vi "cRIO_4DoF_deactivate_mouseforce_axes.vi"(6 "Disable Yaw forces":bool, 8 "Disable X":bool, 9 "Disable Y forces":bool, 10 "Disable -X":bool, 11 "del_m in":dbl[](array[numeric])) -> (3 "del_m out":dbl[](array[numeric]))   [LabVIEW 2019]
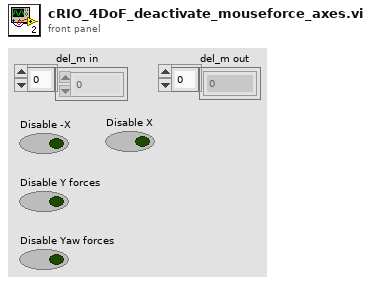
[diagram p1: front panel]
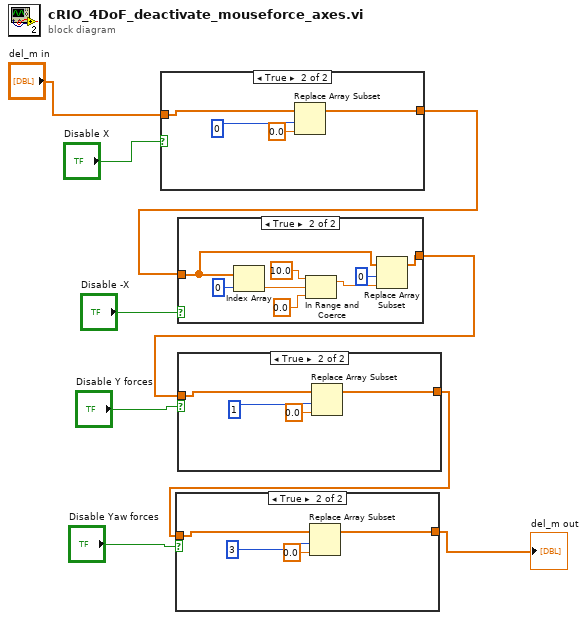
[diagram p0: block diagram]
diagram:
  n1 = case shown="True" "Disable X" {
    tunnel: "del_m in" -> [w10 w14]
    tunnel: [w10 w11] -> w2
    frame False {
    }
    frame True {
      n2 = Replace Array Subset(array=w14, new element=0.0 ("new element/subarray"), index=0) -> (w11:dbl[])
    }
  }
  n3 = case shown="True" "Disable -X" {
    tunnel: w2 -> [w15 w17]
    tunnel: [w15 w16] -> w5
    frame False {
    }
    frame True {
      n4 = Index Array(array=w17, index=0) -> (element=w22:dbl)
      n5 = In Range and Coerce(upper limit=10.0, x=w22, lower limit=0.0) -> (coerced(x)=w19:dbl)  [unwired: 1 out]
      n6 = Replace Array Subset(array=w17, new element=w19, index=0) -> (w16:dbl[])
    }
  }
  n7 = case shown="True" "Disable Y forces" {
    tunnel: w5 -> [w24 w28]
    tunnel: [w24 w25] -> w8
    frame False {
    }
    frame True {
      n8 = Replace Array Subset(array=w28, new element=0.0 ("new element/subarray"), index=1) -> (w25:dbl[])
    }
  }
  n9 = case shown="True" "Disable Yaw forces" {
    tunnel: w8 -> [w29 w33]
    tunnel: [w29 w30] -> w9
    frame False {
    }
    frame True {
      n10 = Replace Array Subset(array=w33, new element=0.0 ("new element/subarray"), index=3) -> (w30:dbl[])
    }
  }
  "del_m out" <- w9
